vi "Choreo_SwerveSample_New.vi"(0 "heading":dbl, 1 "velocityX":dbl, 2 "velocityY":dbl, 3 "angularVelocity":dbl, 4 "accelX":dbl, 5 "accelY":dbl, 6 "y":dbl, 7 "accelAngular":dbl, 8 "x":dbl, 9 "forceX":dbl[](array[numeric]), 10 "timestamp":dbl, 11 "forceY":dbl[](array[numeric])) -> (14 "ChoreoSwerveSample":T1)   [LabVIEW 2019, in "ChoreoLib.lvlib"]
doc: "Constructs a SwerveSample with the specified parameters.\nInputs: \n - timestamp - double - The timestamp of this sample, relative to the beginning of the trajectory.\n - x - double - The X position of the sample in meters.\n - y - double - The Y position of the sample in meters.\n - heading - double - The heading of the sample in radians, with 0 being in the +X direction.\n - velocityX - double - The velocity of the sample in the X direction in m/s.\n - velocityY - double - The velocity of the sample in the Y direction in m/s.\n - angularVelocity - double - The angular velocity of the sample in rad/s.\n - accelX - double - The acceleration of the sample in the X direction in m/s².\n - accelY - double - The acceleration of the sample in the Y direction in m/s².\n - accelAngular - double - The angular acceleration of the sample in rad/s².\n - ForcesX - double array - The force on each swerve module in the X direction in Newtons. Module forces appear in the following order: [FL, FR, BL, BR].\n - ForcesY - double array - The force on each swerve module in the Y direction in Newtons. Module forces appear in the following order: [FL, FR, BL, BR].\n\nOutputs:\n - ChoreoSwerveSample - cluster - Cluster containing sample data"
uses:
  ChoreoLib.lvlib
  TypeDef/ChoreoSwerveSample.ctl
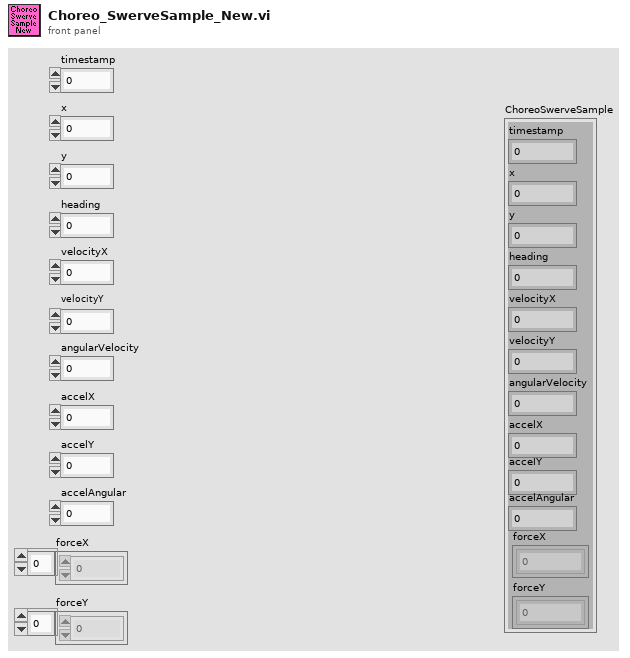
[diagram p1: front panel]
types:
  T1 = typedef "ChoreoLib.lvlib/ChoreoSwerveSample.ctl" = cluster{"timestamp":dbl, "x":dbl, "y":dbl, "heading":dbl, "velocityX":dbl, "velocityY":dbl, "angularVelocity":dbl, "accelX":dbl, "accelY":dbl, "accelAngular":dbl, "forceX":dbl[], "forceY":dbl[]}
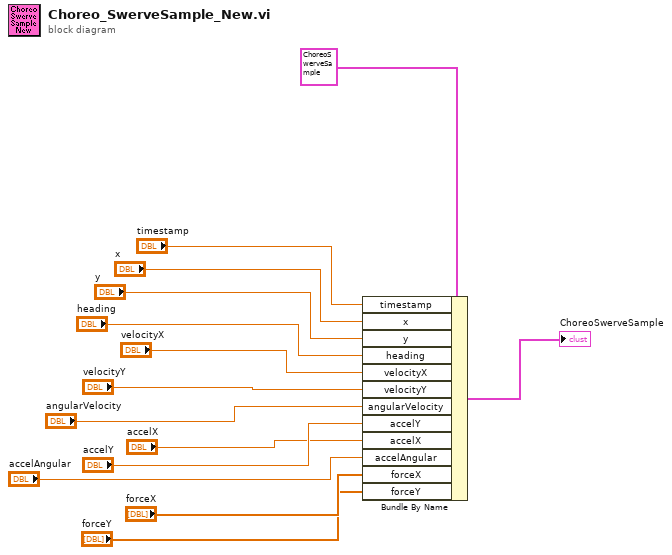
[diagram p0: block diagram]
diagram:
  n1 = Bundle By Name(cluster=T1 {"timestamp"=0.0, "x"=0.0, "y"=0.0, "heading"=0.0, "velocityX"=0.0, "velocityY"=0.0, "angularVelocity"=0.0, "accelX"=0.0, "accelY"=0.0, "accelAngular"=0.0, "forceX"=[], "forceY"=[]} ("ChoreoSwerveSample 2"), "timestamp"="timestamp", "x"="x", "y"="y", "heading"="heading", "velocityX"="velocityX", "velocityY"="velocityY", "angularVelocity"="angularVelocity", "accelY"="accelY", "accelX"="accelX", "accelAngular"="accelAngular", "forceX"="forceX", "forceY"="forceY") -> (→"ChoreoSwerveSample":T1)
